vi "PicoScope2000aOpen.vi"(5 "Serial Number":string, 7 "Use Serial Number":bool, 8 "error in (no error)":errorcluster, 9 "Mode":u16(ring) items=["Dialog On Error", "no dialog - CloseUnit and Stop", "no dialog - Continue", "no dialog - Stop"]) -> (0 "error out":errorcluster, 1 "Max Adc value":i16, 2 "Device Info":T1, 3 "handle":i16, 4 "Pico 2000a Units":string, 6 "serialLth":i16)   [LabVIEW 2010]
doc: "This VI opens a PicoScope 3000a/b and returns a handle to the device."
uses:
  ps2000a.dll
panel:
  out "count":i16
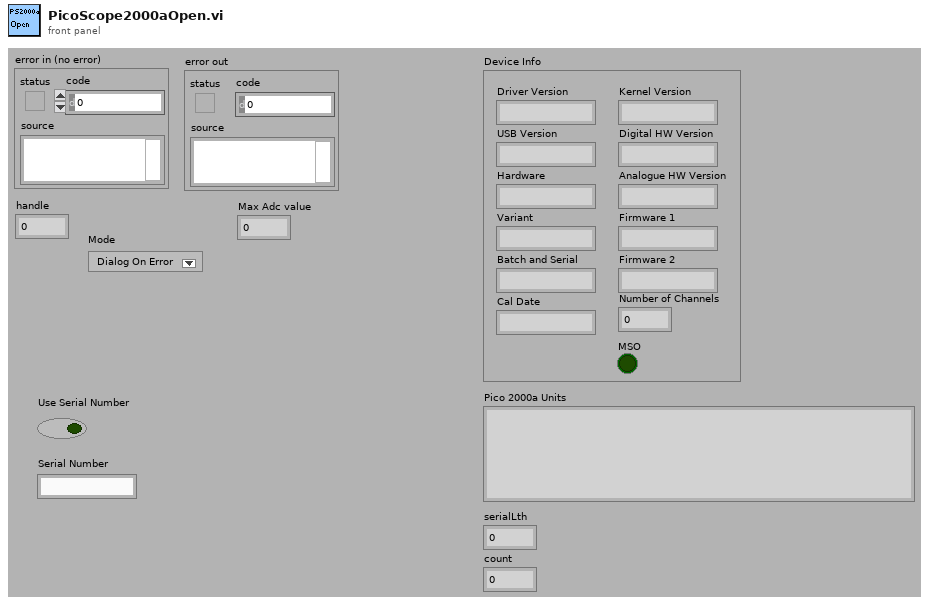
[diagram p1: front panel]
types:
  T1 = cluster{"Driver Version":string, "USB Version":string, "Hardware":string, "Variant":string, "Batch and Serial":string, "Cal Date":string, "Kernel Version":string, "Digital HW Version":string, "Analogue HW Version":string, "Firmware 1":string, "Firmware 2":string, "MSO":bool, "Number of Channels":i16}
  T2 = cluster{"status":bool, "code":u32, "source":string}
  T3 = cluster{"Driver Version":string, "USB Version":string, "Hardware":string, "Variant":string, "Batch and Serial":string, "Cal Date":string, "Kernel Version":string, "Digital HW Version":string, "Analogue HW Version":string, "Firmware 1":string, "Firmware 2":string}
  T4 = cluster{"Driver Version":string, "USB Version":string, "Hardware":string, "Variant":string, "Batch and Serial":string, "Cal Date":string, "Kernel Version":string, "Digital HW Version":string, "Analogue HW Version":string, "Firmware 1":string, "Firmware 2":string, bool, i16}
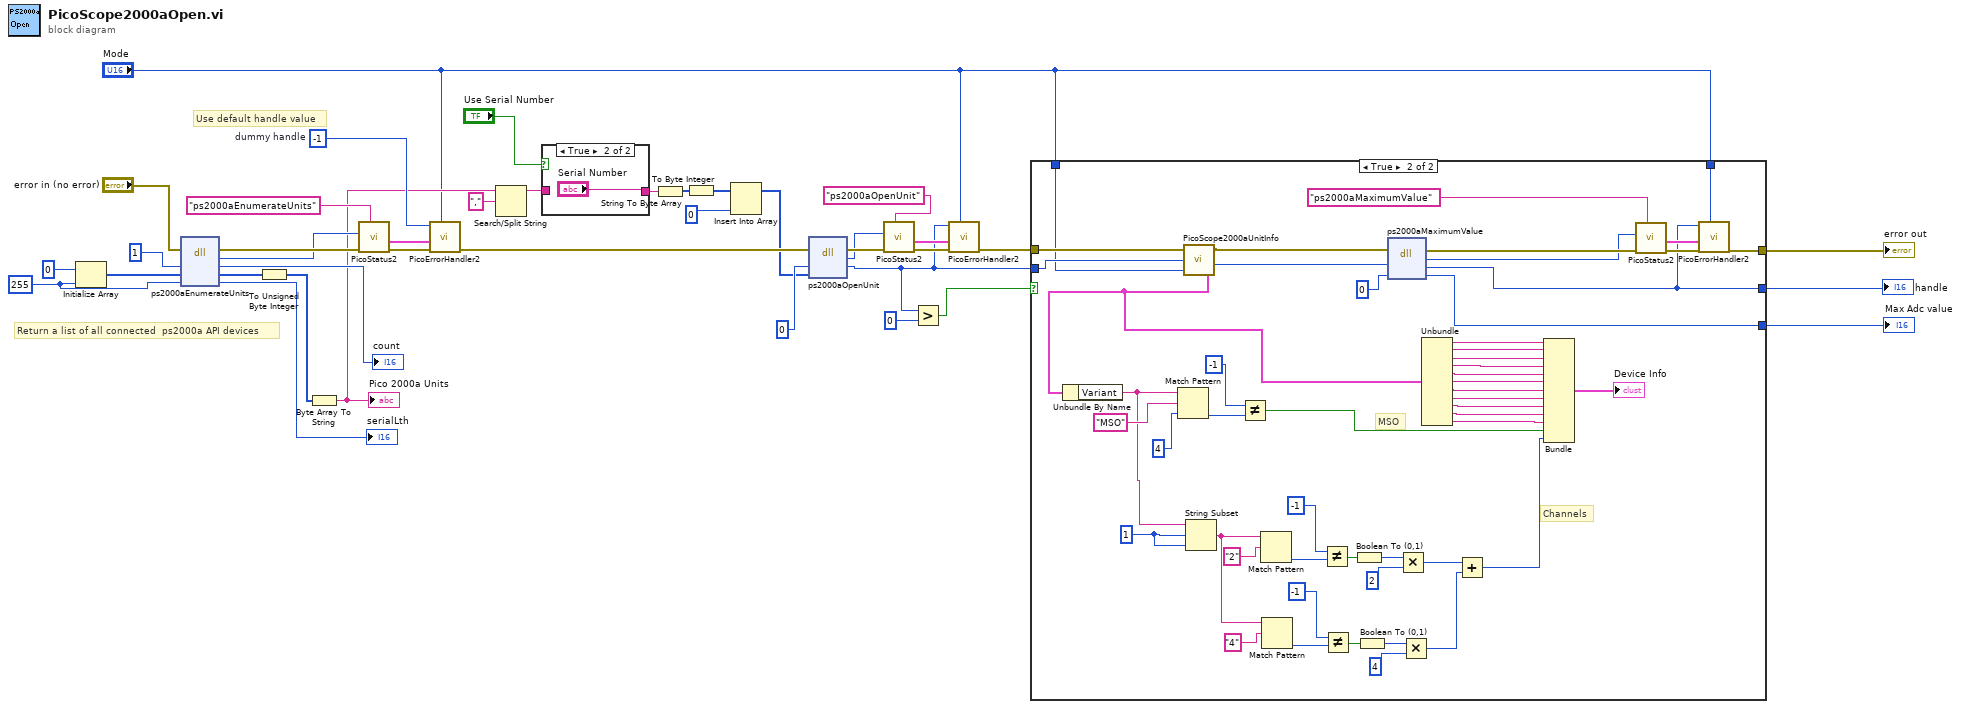
[diagram p0: block diagram]
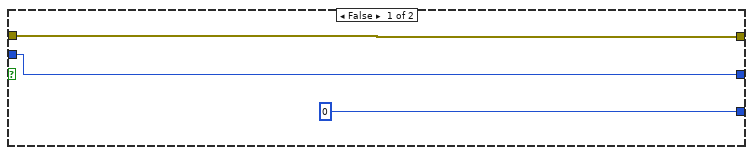
[diagram p3: hidden frame]
diagram:
  w27 = i16 -1  # dummy handle
  w30 = i16 255 ("dimension size")
  # "Use default handle value"
  # "Return a list of all connected  ps2000a API devices"
  n1 = Initialize Array(i8 0 ("U8"), w30) -> (w32:i8[])
  n2 = dll-call lib="ps2000a.dll" fn="ps2000aEnumerateUnits"(error in="error in (no error)", "count"=i16 1, "serials"=w32, "serialLth"=w30) -> (error out=w24:errorcluster, "PICO_STATUS"=w22:u32, "count"=→"count":i16, "serials"=w28:i8[], "serialLth"=→"serialLth":i16)  [unwired: 2 in, 1 out]
  n3 = To Unsigned Byte Integer(number=w28) -> (unsigned 8bit integer=w29:u8[])
  n4 = Byte Array To String(unsigned byte array=w29) -> (string=w20:string)
  "Pico 2000a Units" <- w20
  n5 = call "PicoStatus2.vi"("PICO source"="ps2000aEnumerateUnits" ("source"), "Error in"=w24, "PICO STATUS"=w22) -> ("error out"=w26:errorcluster, "PICO_STATUS out"=w25:T2)  [unwired: 5 in]
  n6 = call "PicoErrorHandler2.vi"("Mode"="Mode", "error in (no error)"=w26, "PICO_STATUS in"=w25, "handle In"=w27) -> ("error out"=w11:errorcluster)  [unwired: 7 in]
  n7 = Search/Split String(string=w20, search string/char (-)=",") -> (substring before match=w18:string)  [unwired: 1 in, 2 out]
  n8 = case shown="True" "Use Serial Number" {
    tunnel: w18 -> [w40 _]
    tunnel: [w40 "Serial Number"] -> w14
    frame False {
    }
    frame True {
    }
  }
  n9 = String To Byte Array(string=w14) -> (unsigned byte array=w16:u8[])
  n10 = To Byte Integer(number=w16) -> (8bit integer=w17:i8[])
  n11 = Insert Into Array(array=w17, new element=i8 0 ("new element/subarray")) -> (w10:i8[])  [unwired: 1 in]
  n12 = dll-call lib="ps2000a.dll" fn="ps2000aOpenUnit" ("ps3000.dll:_ps3000_open_unit@0")(error in=w11, "handle"=i16 0, "serial"=w10) -> (error out=w8:errorcluster, "PICO_STATUS"=w7:u32, "handle"=w3:i16)  [unwired: 3 in, 1 out]
  n13 = call "PicoStatus2.vi"("PICO source"="ps2000aOpenUnit" ("source"), "Error in"=w8, "PICO STATUS"=w7) -> ("error out"=w9:errorcluster, "PICO_STATUS out"=w5:T2)  [unwired: 5 in]
  n14 = Greater?(x=w3, y=i16 0) -> (0:w39:bool)
  n15 = call "PicoErrorHandler2.vi"("Mode"="Mode", "error in (no error)"=w9, "PICO_STATUS in"=w5, "handle In"=w3) -> ("error out"=w4:errorcluster)  [unwired: 7 in]
  n16 = case shown="True" w39 {
    tunnel: w3 -> [w43 w94]
    tunnel: w4 -> [w44 w95]
    tunnel: [w44 w47] -> w1
    tunnel: [w43 w45] -> w36
    tunnel: [i16 0 ("value") w93] -> w37
    tunnel: "Mode" -> [_ w50]
    tunnel: "Mode" -> [_ w49]
    frame False {
    }
    frame True {
      w74 = 1 ("offset (0)")
      # "MSO"
      # "Channels"
      n17 = call "PicoScope2000aUnitInfo.vi"("error in (no error)"=w95, "handle in"=w94, "Mode"=w50) -> ("error out"=w54:errorcluster, "handle out"=w55:i16, "Unit Info"=w86:T3)  [unwired: 1 out]
      n18 = Unbundle By Name(w86) -> ("Variant"=w58:string)
      n19 = Match Pattern(string=w58, regular expression="MSO", offset (0)=4) -> (offset past match=w90:i32)  [unwired: 3 out]
      n20 = String Subset(string=w58, offset (0)=w74, length (rest)=w74) -> (substring=w67:string)
      n21 = Not Equal?(x=-1, y=w90) -> (x != y?=w87:bool)
      n22 = Match Pattern(string=w67, regular expression="2") -> (offset past match=w72:i32)  [unwired: 1 in, 3 out]
      n23 = Match Pattern(string=w67, regular expression="4") -> (offset past match=w69:i32)  [unwired: 1 in, 3 out]
      n24 = Not Equal?(x=-1, y=w72) -> (x != y?=w64:bool)
      n25 = Not Equal?(x=-1, y=w69) -> (x != y?=w60:bool)
      n26 = Boolean To (0,1)(Boolean=w64) -> (0, 1=w63:i16)
      n27 = Boolean To (0,1)(Boolean=w60) -> (0, 1=w61:i16)
      n28 = dll-call lib="ps2000a.dll" fn="ps2000aMaximumValue"(error in=w54, "handle"=w55, "value"=i16 0) -> (error out=w53:errorcluster, "PICO_STATUS"=w52:u32, "handle"=w45:i16, "value"=w93:i16)  [unwired: 2 in, 1 out]
      n29 = Multiply(x=w63, y=i16 2) -> (x*y=w66:i16)
      n30 = Multiply(x=w61, y=i16 4) -> (x*y=w59:i16)
      n31 = Unbundle(w86) -> ("Driver Version"=w75:string, "USB Version"=w76:string, "Hardware"=w77:string, "Variant"=w78:string, "Batch and Serial"=w79:string, "Cal Date"=w80:string, "Kernel Version"=w81:string, "Digital HW Version"=w82:string, "Analogue HW Version"=w83:string, "Firmware 1"=w84:string, "Firmware 2"=w85:string)
      n32 = Add(x=w66, y=w59) -> (x+y=w57:i16)
      n33 = Bundle("Driver Version"=w75, "USB Version"=w76, "Hardware"=w77, "Variant"=w78, "Batch and Serial"=w79, "Cal Date"=w80, "Kernel Version"=w81, "Digital HW Version"=w82, "Analogue HW Version"=w83, "Firmware 1"=w84, "Firmware 2"=w85, w87, w57) -> (→"Device Info":T4)  [unwired: 1 in]
      n34 = call "PicoStatus2.vi"("PICO source"="ps2000aMaximumValue" ("source"), "Error in"=w53, "PICO STATUS"=w52) -> ("error out"=w48:errorcluster, "PICO_STATUS out"=w46:T2)  [unwired: 5 in]
      n35 = call "PicoErrorHandler2.vi"("Mode"=w49, "error in (no error)"=w48, "PICO_STATUS in"=w46, "handle In"=w45) -> ("error out"=w47:errorcluster)  [unwired: 7 in]
    }
  }
  "handle" <- w36
  "error out" <- w1
  "Max Adc value" <- w37
